vi "Make.vi"(8 "error in (no error)":errorcluster, 9 "Item Refnum":refnum<vi>, 10 "Target":refnum<vi>, 11 "Abstract Message Scripter":refnum<class "Abstract Message Scripter.lvclass">) -> (0 "error out":errorcluster, 3 "Abstract Message Scripter out":refnum<class "Abstract Message Scripter.lvclass">)   [LabVIEW 2020, in "Message Maker.lvlib" / "Abstract Message Scripter.lvclass"]
uses:
  Abstract Message Scripter.lvclass
  Abstract Message Scripter.lvclass/Abstract Message Scripter.ctl
  Message Maker.lvlib
  Message Scripter/Message Scripter.lvclass
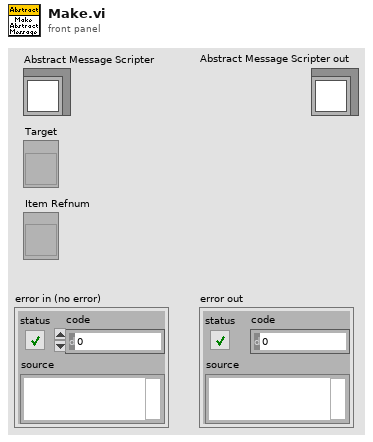
[diagram p1: front panel]
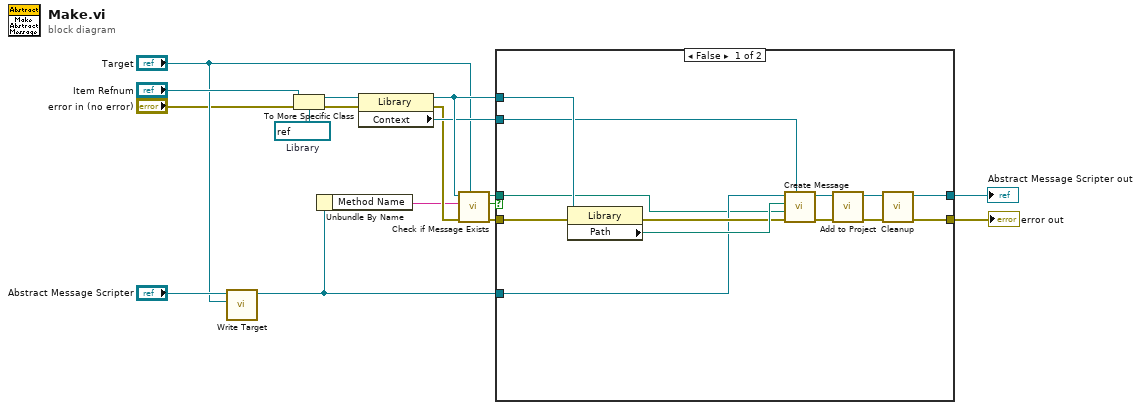
[diagram p0: block diagram]
diagram:
  w10 = refnum<vi> refnum  # Library
  n1 = call "Write Target.vi"("Target"="Target", "Message Scripter in"="Abstract Message Scripter") -> ("Message Scripter out"=w4:refnum<class "Abstract Message Scripter.lvclass">)  [unwired: 9 in]
  n2 = To More Specific Class(target class=w10, reference="Item Refnum", error in="error in (no error)") -> (specific class reference=w8:refnum<vi>, error out=w9:errorcluster)
  n3 = Unbundle By Name(w4) -> ("Method Name"=w6:string)
  n4 = property class="Library"(reference=w8, error in=w9) -> (reference out=w13:refnum<vi>, error out=w11:errorcluster, "Context"=w12:refnum<vi>)
  n5 = call "Check if Message Exists.vi"("Target"="Target", "error in (no error)"=w11, "Method Name"=w6, "Actor"=w13) -> ("error out"=w17:errorcluster, "Message Class Exists?"=w16:bool, "Message Path"=w14:path)  [unwired: 5 in]
  n6 = case shown="False" w16 {
    tunnel: w12 -> [w22 _]
    tunnel: w13 -> [w25 _]
    tunnel: w14 -> [w23 _]
    tunnel: w17 -> [w30 w32]
    tunnel: [w20 w32] -> w15
    tunnel: w4 -> [w24 w31]
    tunnel: [w18 w31] -> w7
    frame False {
      n7 = property class="Library"(reference=w25, error in=w30) -> (error out=w26:errorcluster, "Path"=w27:path)  [unwired: 1 out]
      n8 = call "Create Message.vi"("AppInst"=w22, "error in (no error)"=w26, "Destination Path"=w23, "Actor class path"=w27, "Message Maker in"=w24) -> ("error out"=w28:errorcluster, "Message Maker out"=w29:refnum<class "Abstract Message Scripter.lvclass">)  [unwired: 5 in]
      n9 = call-dynamic "Add to Project.vi"("error in (no error)"=w28, "Abstract Message Scripter in"=w29) -> ("error out"=w21:errorcluster, "Abstract Message Scripter out"=w19:refnum<class "Abstract Message Scripter.lvclass">)  [unwired: 8 in]
      n10 = call-dynamic "Cleanup.vi"("error in (no error)"=w21, "Message Scripter in"=w19) -> ("error out"=w20:errorcluster, "Message Scripter out"=w18:refnum<class "Abstract Message Scripter.lvclass">)  [unwired: 8 in]
    }
    frame True {
    }
  }
  "error out" <- w15
  "Abstract Message Scripter out" <- w7
